vi "IO20 DAQ Control MAIN.vi"(8 "error in (no error)":errorcluster, 11 "IO20 Control Sequencer":T1[](array[typedef])) -> (0 "error out":errorcluster, 3 "ADC Data":T3(array[cluster]))   [LabVIEW 2020, in "DLP Design Modules Driver.lvlib"]
doc: "Developed By: J Branch\nLast Update: 10/9/2022\n\nDescription: Allows user control of the DLP IO20 DAQ module through LabVIEW. This DAQ module is a relatively simple to use programatically configurable USB DAQ device.\n\nSee the datasheet from DLP Design to view more about the device description."
uses:
  DLP Design Modules Driver.lvlib
  IO20_Config1_typedef.ctl
panel:
  in  "Tab Control":enum32{"User", "Back Params"}(tab)
  out "CMD & Responses":T2(array[cluster])
  out "UserMsg":string="Specify DAQ actions to be performed using the IO20 Control Sequencer prior to running the program.\n\n"
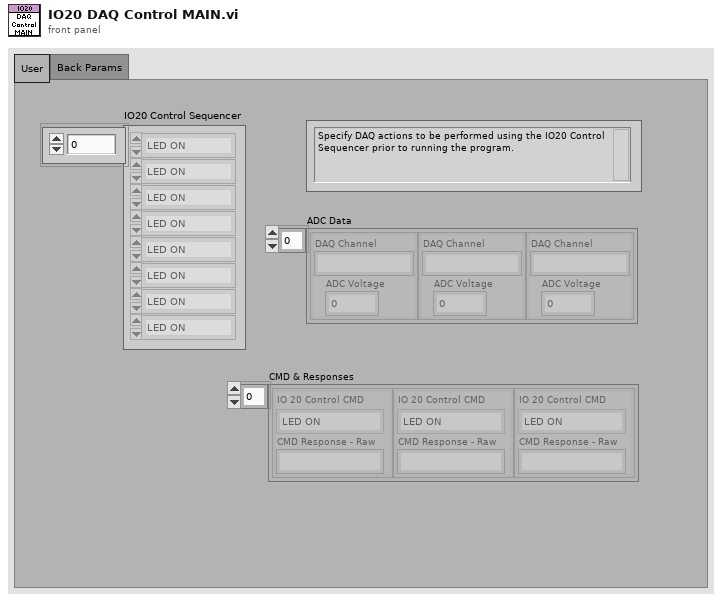
[diagram p1: front panel]
types:
  T1 = typedef "DLP Design Modules Driver.lvlib/IO20_Config1_typedef.ctl" = enum16{"Ping", "Flash LED", "LED OFF", "LED ON", "Relay 1 Set", "Relay 1 Reset", "Relay 2 Set", "Relay 2 Reset", "AN0-DI", "AN1-DI", "AN2-DI", "RB6-DI", "RB7-DI", "AN3-AI", "AN4-AI", "AN5-AI", "AN6-AI", "AN7-AI", "AN8-AI", "AN9-AI", "AN10-AI", "AN11-AI", "AN12-AI", "AN13-AI", "P5-DO-low", "P5-DO-high", "P6-DO-low", "P6-DO-high", "P7-DO-low", "P7-DO-high"}
  T2 = cluster{"IO 20 Control CMD":T1, "CMD Response - Raw":string}[]
  T3 = cluster{"DAQ Channel":string, "ADC Voltage":dbl}[]
  T4 = cluster{"IO 20 Control CMD":T1, "Read Buffer":string}[]
  T5 = cluster{"IO 20 Control CMD":T1, "Read Buffer":string}
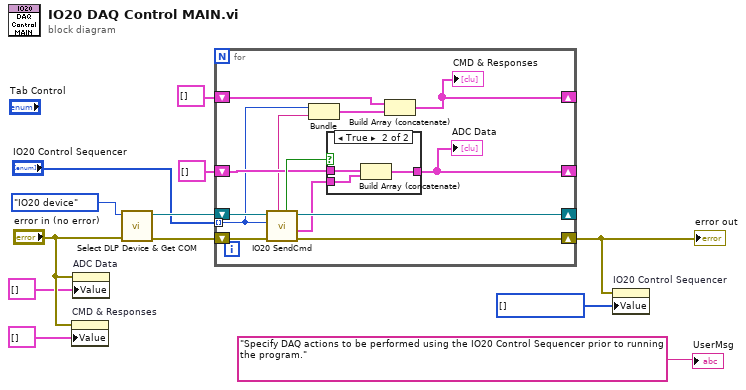
[diagram p0: block diagram]
diagram:
  w5 = T1[] [] items=["Ping", "Flash LED", "LED OFF", "LED ON", "Relay 1 Set", "Relay 1 Reset", "Relay 2 Set", "Relay 2 Reset", "AN0-DI", "AN1-DI", "AN2-DI", "RB6-DI", "RB7-DI", "AN3-AI", "AN4-AI", "AN5-AI", "AN6-AI", "AN7-AI", "AN8-AI", "AN9-AI", "AN10-AI", "AN11-AI", "AN12-AI", "AN13-AI", "P5-DO-low", "P5-DO-high", "P6-DO-low", "P6-DO-high", "P7-DO-low", "P7-DO-high"] ("IO20 Control Sequencer")
  n1 = property on="CMD & Responses" class="Arr (strict)"(error in="error in (no error)", "Value"=T2 [] ("CMD & Responses")) -> ()  [unwired: 1 in, 2 out]
  n2 = property on="ADC Data" class="Arr (strict)"(error in="error in (no error)", "Value"=T3 [] ("ADC Data")) -> ()  [unwired: 1 in, 2 out]
  n3 = call "Select DLP Device & Get COM.vi"("error in (no error)"="error in (no error)", "Device Type Selection"=enum16{"IOR4 device", "IO20 device"}."IO20 device") -> ("error out"=w11:errorcluster, "Selected COM"=w12:refnum<visa-resource-name>)  [unwired: 7 in, 1 out]
  n4 = for {
    shift-right: [w23] -> w6
    shift-left: w11 -> [w24]
    tunnel: "IO20 Control Sequencer" -> [w15] mode=indexing
    shift-right: [w21] -> _
    shift-left: w12 -> [w25]
    shift-right: [w18] -> _
    shift-left: T3 [] -> [w19]
    shift-right: [w13] -> _
    shift-left: T4 [] -> [w14]
    n5 = call "IO20 SendCmd.vi"("error in"=w24, "CMD"=w15, "IO20 VISA"=w25) -> ("error out"=w23:errorcluster, "ADC Data Out"=w20:cluster{"DAQ Channel":string, "ADC Voltage":dbl}, "IO20 VISA-OUT"=w21:refnum<visa-resource-name>, "ADC Volt"=w22:bool, "Read Buffer"=w17:string)  [unwired: 3 in, 1 out]
    n6 = Bundle("IO 20 Control CMD"=w15, "Read Buffer"=w17) -> (w16:T5)  [unwired: 1 in]
    n7 = case shown="True" w22 {
      tunnel: [w26 w29] -> w18
      tunnel: w20 -> [_ w28]
      tunnel: w19 -> [w26 w27]
      frame False {
      }
      frame True {
        n8 = Build Array (concatenate)(w27, w28) -> (w29:T3)
      }
    }
    "ADC Data" <- w18
    n9 = Build Array (concatenate)(w14, w16) -> (w13:T4)
    "CMD & Responses" <- w13
  }
  "error out" <- w6
  n10 = property on="IO20 Control Sequencer" class="Arr (strict)"(error in=w6, "Value"=w5) -> ()  [unwired: 1 in, 2 out]
  "UserMsg" <- "Specify DAQ actions to be performed using the IO20 Control Sequencer prior to running the program." ("UserMsg")
